vi "ResolveOrUseCachedURL.vi"(8 "error in (no error)":errorcluster, 10 "Cached Resolved URL":string, 11 "Unresolved URL":string) -> (0 "error out":errorcluster, 2 "Unresolved URL out":string, 3 "Resolved URL out":string)   [LabVIEW 2017]
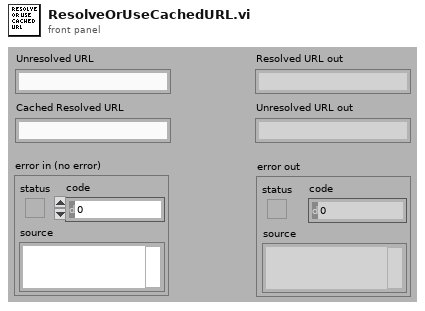
[diagram p1: front panel]
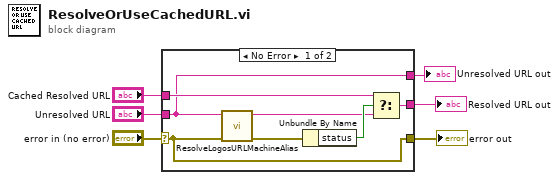
[diagram p0: block diagram]
diagram:
  n1 = case shown="No Error" "error in (no error)" {
    selector: "error in (no error)" -> [w10 w15]
    tunnel: "Unresolved URL" -> [w8 w14]
    tunnel: [w13 w14] -> w2
    tunnel: "Cached Resolved URL" -> [w9 _]
    tunnel: [w10 w15] -> w5
    tunnel: [w8 w14] -> w1
    frame No Error {
      n2 = call <vilib>:"ResolveLogosURLMachineAlias.vi"("error in (no error)"=w10, "Unresolved URL"=w8) -> ("error out"=w12:errorcluster, "Resolved URL"=w7:string)  [unwired: 8 in]
      n3 = Unbundle By Name(w12) -> ("status"=w11:bool)
      n4 = Select(t=w9, s=w11, f=w7) -> (s? t:f=w13:string)
    }
    frame Error {
    }
  }
  "Resolved URL out" <- w2
  "error out" <- w5
  "Unresolved URL out" <- w1
